vi "读取寄存器新.vi"(7 "VISA Resource":refnum<visa-resource-name>, 9 "Slave ID":u8=1, 10 "quantity":u16, 11 "starting address":u16) -> (0 "Registers":u16[](array[numeric]))   [LabVIEW 2016]
uses:
  <vilib>/Plasmionique/MB Master/MB_Master_Serial/MB_Master_Serial.lvclass
  F:/Program Files/National Instruments/LabVIEW 2016/vi.lib/Plasmionique/MB Master/MB_Master/MB_Master.lvclass
  <vilib>/Plasmionique/MB Master/MB Master.lvlib
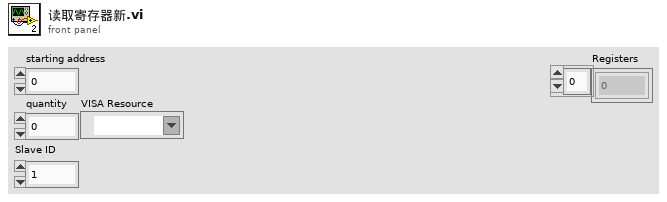
[diagram p1: front panel]
types:
  T1 = cluster{"baud rate (bps)":u32, "stop bits":u16, "parity":u16, "flow control":u16, "timeout":u32, "retries":i32}
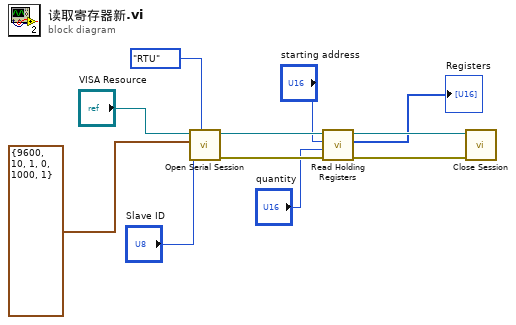
[diagram p0: block diagram]
diagram:
  n1 = call <vilib>:"Open Serial Session.vi"("Mode (RTU)"=enum16{"RTU", "ASCII"}."RTU", "Slave ID"="Slave ID", "Serial Config"=T1 {"baud rate (bps)"=9600, "stop bits"=10, "parity"=1, "flow control"=0, "timeout"=1000, "retries"=1}, "VISA Resource"="VISA Resource") -> ("Error out"=w8:errorcluster, "MB_Serial session"=w11:refnum<class "MB_Master_Serial.lvclass">)  [unwired: 6 in]
  n2 = call <vilib>:"Read Holding Registers.vi"("error in (no error)"=w8, "quantity"="quantity", "starting address"="starting address", "MB session in"=w11) -> ("error out"=w9:errorcluster, "Registers"=→"Registers":u16[], "MB session out"=w10:refnum<class "MB_Master_Serial.lvclass">)  [unwired: 5 in]
  n3 = call-dynamic "Close Session.vi"("error in (no error)"=w9, "MB_Serial session"=w10) -> ()  [unwired: 9 in, 1 out]
